vi "arrayDoppelMoppel-11-15.vi"(8 "verdoppeln":i32[](array[numeric]), 9 "Traps/MachsKoeff2":dbl[](array[numeric]), 10 "Traps/MachsKoeff1":dbl[](array[numeric]), 11 "Traps/MachsKoeff0":dbl[](array[numeric])) -> (1 "Traps/MachsKoeff2":dbl[](array[numeric]), 2 "Traps/MachsKoeff1":dbl[](array[numeric]), 3 "Traps/MachsKoeff0":dbl[](array[numeric]))   [LabVIEW 2010]
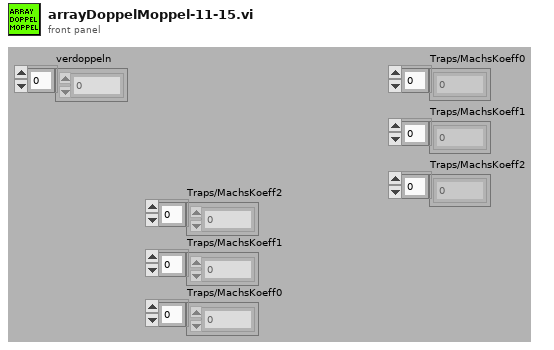
[diagram p1: front panel]
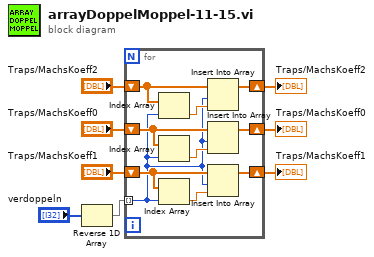
[diagram p0: block diagram]
diagram:
  n1 = Reverse 1D Array(array="verdoppeln") -> (reversed array=w4:i32[])
  n2 = for {
    tunnel: w4 -> [w11] mode=indexing
    shift-right: [w16] -> w3
    shift-left: "Traps/MachsKoeff0" -> [w17]
    shift-right: [w12] -> w2
    shift-left: "Traps/MachsKoeff1" -> [w13]
    shift-right: [w9] -> w1
    shift-left: "Traps/MachsKoeff2" -> [w10]
    n3 = Index Array(array=w10, index=w11) -> (element=w14:dbl)
    n4 = Index Array(array=w17, index=w11) -> (element=w18:dbl)
    n5 = Index Array(array=w13, index=w11) -> (element=w15:dbl)
    n6 = Insert Into Array(array=w10, index=w11, new element=w14) -> (w9:dbl[])
    n7 = Insert Into Array(array=w17, index=w11, new element=w18) -> (w16:dbl[])
    n8 = Insert Into Array(array=w13, index=w11, new element=w15) -> (w12:dbl[])
  }
  "Traps/MachsKoeff0" <- w3
  "Traps/MachsKoeff1" <- w2
  "Traps/MachsKoeff2" <- w1
